vi "Global LM model function and gradient (1-Exp, Convolved, Periodic).vi"(3 "output control":T1, 4 "data":variant, 5 "X":dbl[](array[numeric]), 6 "a":dbl[](array[numeric])) -> (0 "error out":errorcluster, 1 "f'(X,a)":dbl[][](array[numeric]), 2 "f(X,a)":dbl[](array[numeric]))   [LabVIEW 2021, in "Fits.lvlib"]
doc: "This template is the starting point for creating a model function to be passed to the Nonlinear Curve Fit.vi."
uses:
  <vilib>/gmath/NumericalOptimization/LM_output select.ctl
  Global Fits/Global Fit Data.ctl
  Global Fits/Global Fit Parameters Information.ctl
  Fits.lvlib
  <vilib>/gmath/NI_Gmath.lvlib
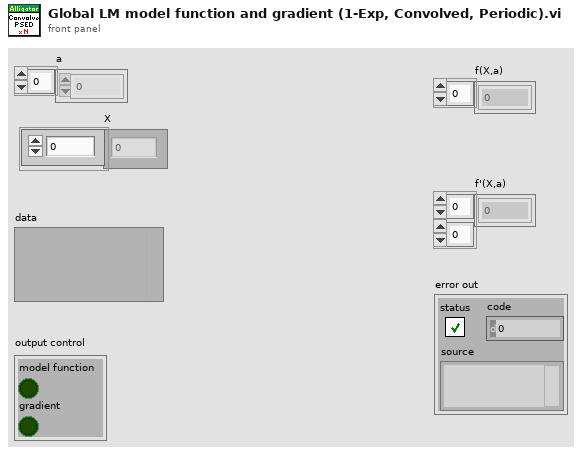
[diagram p1: front panel]
types:
  T1 = typedef "NI_Gmath.lvlib/LM_output select.ctl" = cluster{"model function":bool, "gradient":bool}
  T2 = typedef "Global Fit Data.ctl" = cluster{"Fit Data":variant, "Global Fit Parameter Information":T3, "# Points in Plots":i32[]}
  T3 = typedef "Fits.lvlib/Global Fit Parameters Information.ctl" = cluster{"Original Parameter Indices":i32[], "# Global Parameters":i32, "# Plot Specific Parameters":i32, "Global Parameter? Array":bool[]}
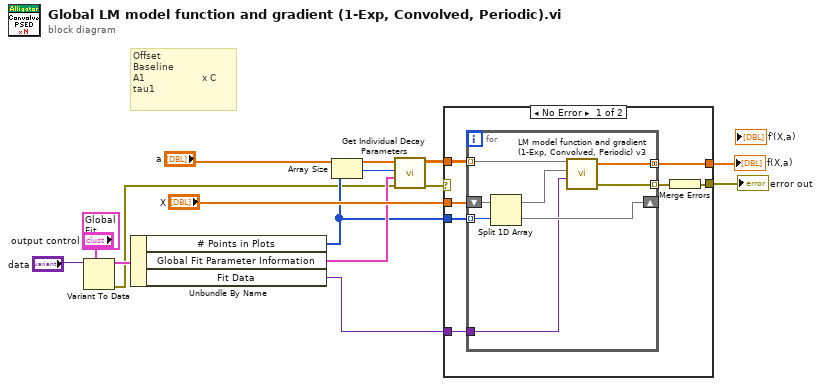
[diagram p0: block diagram]
diagram:
  # "Offset \nBaseline\nA1                   x C\ntau1"
  n1 = Variant To Data(type=T2 {"Fit Data"=variant(cluster{"t Array":dbl[], "IRF Array":dbl[]} {"t Array"=[], "IRF Array"=[]}), "Global Fit Parameter Information"={"Original Parameter Indices"=[], "# Global Parameters"=0, "# Plot Specific Parameters"=0, "Global Parameter? Array"=[]}, "# Points in Plots"=[]} ("IRF"), Variant="data") -> (data=w11:T2, error out=w7:errorcluster)  [unwired: 1 in]
  n2 = Unbundle By Name(w11) -> ("# Points in Plots"=w8:i32[], "Global Fit Parameter Information"=w9:T3, "Fit Data"=w3:variant)
  n3 = Array Size(array=w8) -> (size(s)=w5:i32)
  n4 = call "Get Individual Decay Parameters.vi"("Error In"=w7, "Global Fit Parameter Info"=w9, "# Decays"=w5, "Global Fit Parameters Array"="a") -> ("Error Out"=w4:errorcluster, "All Parameters Array"=w6:dbl[][])  [unwired: 4 in, 2 out]
  n5 = case shown="No Error" w4 {
    selector: w4 -> [_ w30]
    tunnel: "X" -> [w21 _]
    tunnel: w8 -> [w20 _]
    tunnel: w6 -> [w19 _]
    tunnel: w3 -> [w18 _]
    tunnel: [w17 _] -> w2
    tunnel: [w15 w30] -> w1
    frame No Error {
      n6 = for {
        tunnel: w19 -> [w26] mode=indexing
        shift-right: [w27] -> _
        shift-left: w21 -> [w29]
        tunnel: w20 -> [w28] mode=indexing
        tunnel: w18 -> [w24]
        tunnel: [w23] -> w17 mode=concatenating
        tunnel: [w22] -> w16 mode=indexing
        n7 = Split 1D Array(array=w29, index=w28) -> (first subarray=w25:dbl[], second subarray=w27:dbl[])
        n8 = call "LM model function and gradient (1-Exp, Convolved, Periodic) v3.vi"("data"=w24, "X"=w25, "a"=w26) -> ("error out"=w22:errorcluster, "f(X,a)"=w23:dbl[])  [unwired: 1 in, 1 out]
      }
      n9 = Merge Errors(w16) -> (w15:errorcluster)
    }
    frame Error {
    }
  }
  "f(X,a)" <- w2
  "error out" <- w1
